vi "Settings Dialog.vi"(8 "error in (no error)":errorcluster, 11 "Settings in":T2={"Hardware Configuration"={"DAQmx Channel"="", "Max Input"=10.0, "Min Input"=-10.0, "Sample Rate"=1000.0, "DAQmx Task"=""}, "Logging Configuration"={"Log File Base Path"=path "", "TDMS File Reference"=refnum, "Samples to Save"=0, "Trigger - Time"=0, "Trigger - Threshold"=0.0, "Trigger - Channel"=0, "Enable Time Trigger"=FALSE, "Enable Threshold Trigger"=FALSE, "Always Log"=FALSE}, "MSpeed AO HW Config"={"MSpeed AO Channel"="", "Sample Rate(Hz)"=1000.0, "MSpeed AO Task"=""}, "Motor Config"={"VISA resource name"="", "Speed and Duration"=[{"Speed (%)"=10, "Duration (sec)"=120.0}, {"Speed (%)"=25, "Duration (sec)"=120.0}, {"Speed (%)"=50, "Duration (sec)"=120.0}]}, "2P Trigger Config"={"DO Line"="Dev1/port0/line0"}} {"Motor Config"."Speed and Duration"."Duration (sec)" min=0.0 max=100.0 step=0.1 format="%.1f"; "Motor Config"."Speed and Duration"."Speed (%)" min=0 max=100 step=1 format="%.1f"}) -> (0 "error out":errorcluster, 1 "Cancelled?":bool=TRUE, 2 "UI Refresh Needed?":bool, 3 "Settings out":T2={"Hardware Configuration"={"DAQmx Channel"="", "Max Input"=10.0, "Min Input"=-10.0, "Sample Rate"=1000.0, "DAQmx Task"=""}, "Logging Configuration"={"Log File Base Path"=path "C:/Users/jpassiak/Documents/LabVIEW Data/Logged Data.tdms", "TDMS File Reference"=refnum, "Samples to Save"=0, "Trigger - Time"=0, "Trigger - Threshold"=0.0, "Trigger - Channel"=0, "Enable Time Trigger"=FALSE, "Enable Threshold Trigger"=FALSE, "Always Log"=FALSE}, "MSpeed AO HW Config"={"MSpeed AO Channel"="", "Sample Rate(Hz)"=1000.0, "MSpeed AO Task"=""}, "Motor Config"={"VISA resource name"="", "Speed and Duration"=[{"Speed (%)"=10, "Duration (sec)"=120.0}, {"Speed (%)"=25, "Duration (sec)"=120.0}, {"Speed (%)"=50, "Duration (sec)"=120.0}]}, "2P Trigger Config"={"DO Line"="Dev1/port0/line0"}} {"Motor Config"."Speed and Duration"."Duration (sec)" min=0.0 max=100.0 step=0.1 format="%.1f"; "Motor Config"."Speed and Duration"."Speed (%)" min=0 max=100 step=1 format="%.1f"})   [LabVIEW 2016, in "Settings.lvlib"]
doc: "Dialog for selecting user specified settings."
uses:
  Settings.lvlib
  Settings.ctl
  Acquisition/Hardware Configuration.ctl
  Logging/Logging Configuration.ctl
  Motor Speed/MSpeed AO HW Config.ctl
  Motor Control/Motor Control Config.ctl
  Motor Control/Speed and Duration.ctl
  2P Trigger/2P Trigger Config.ctl
  <vilib>/Utility/xml.llb/Write to XML File(string).vi
  Acquisition/Acquisition.lvlib
  Logging/Logging.lvlib
  Motor Speed/Motor Speed AO.lvlib
  Motor Control/Motor Control.lvlib
  2P Trigger/2P Trigger.lvlib
panel:
  in  "Trigger Input DO Line":tag="Dev1/port0/line0"
  in  "VISA resource name":refnum<visa-resource-name>="COM3"
  in  "Speed and Duration":T1[](array[typedef])=[{"Speed (%)"=10, "Duration (sec)"=120.0}, {"Speed (%)"=25, "Duration (sec)"=120.0}, {"Speed (%)"=50, "Duration (sec)"=120.0}] {"Duration (sec)" min=0.0 max=100.0 step=0.1 format="%.1f"; "Speed (%)" min=0 max=100 step=1 format="%.1f"}
  in  "MSpeed Sample Rate":dbl=1000.0
  in  "MSpeed AO Channel":tag="Dev2/ao0"
  in  "Log when triggered":bool
  in  "Trigger Channel":u32
  in  "Samples to Log":u32=500 min=1
  in  "Trigger Threshold (V)":dbl=2.0
  in  "Trigger Time (min)":u32=1
  in  "Enable Threshold Trigger (V):":bool
  in  "Enable Time Trigger (min):":bool
  in  "Always Log":bool=TRUE
  in  "Sample Rate":dbl=1000.0
  in  "Minimum Input":dbl=-10.0
  in  "Maximum Input":dbl=10.0
  in  "DAQmx Channel":tag="Dev1/ai0"
  in  "Log File Path":path
  in  "Cancel Button":bool
  in  "OK Button":bool
  # "Acquisition"
  # "Motor"
  # "Non visible portion of dialog (needed for connector pane)."
  # "Speed (%)"
  # "Duration (sec)"
  # "Trigger"
  # "Speed monitor"
  # "2P trigger"
  # "Logging"
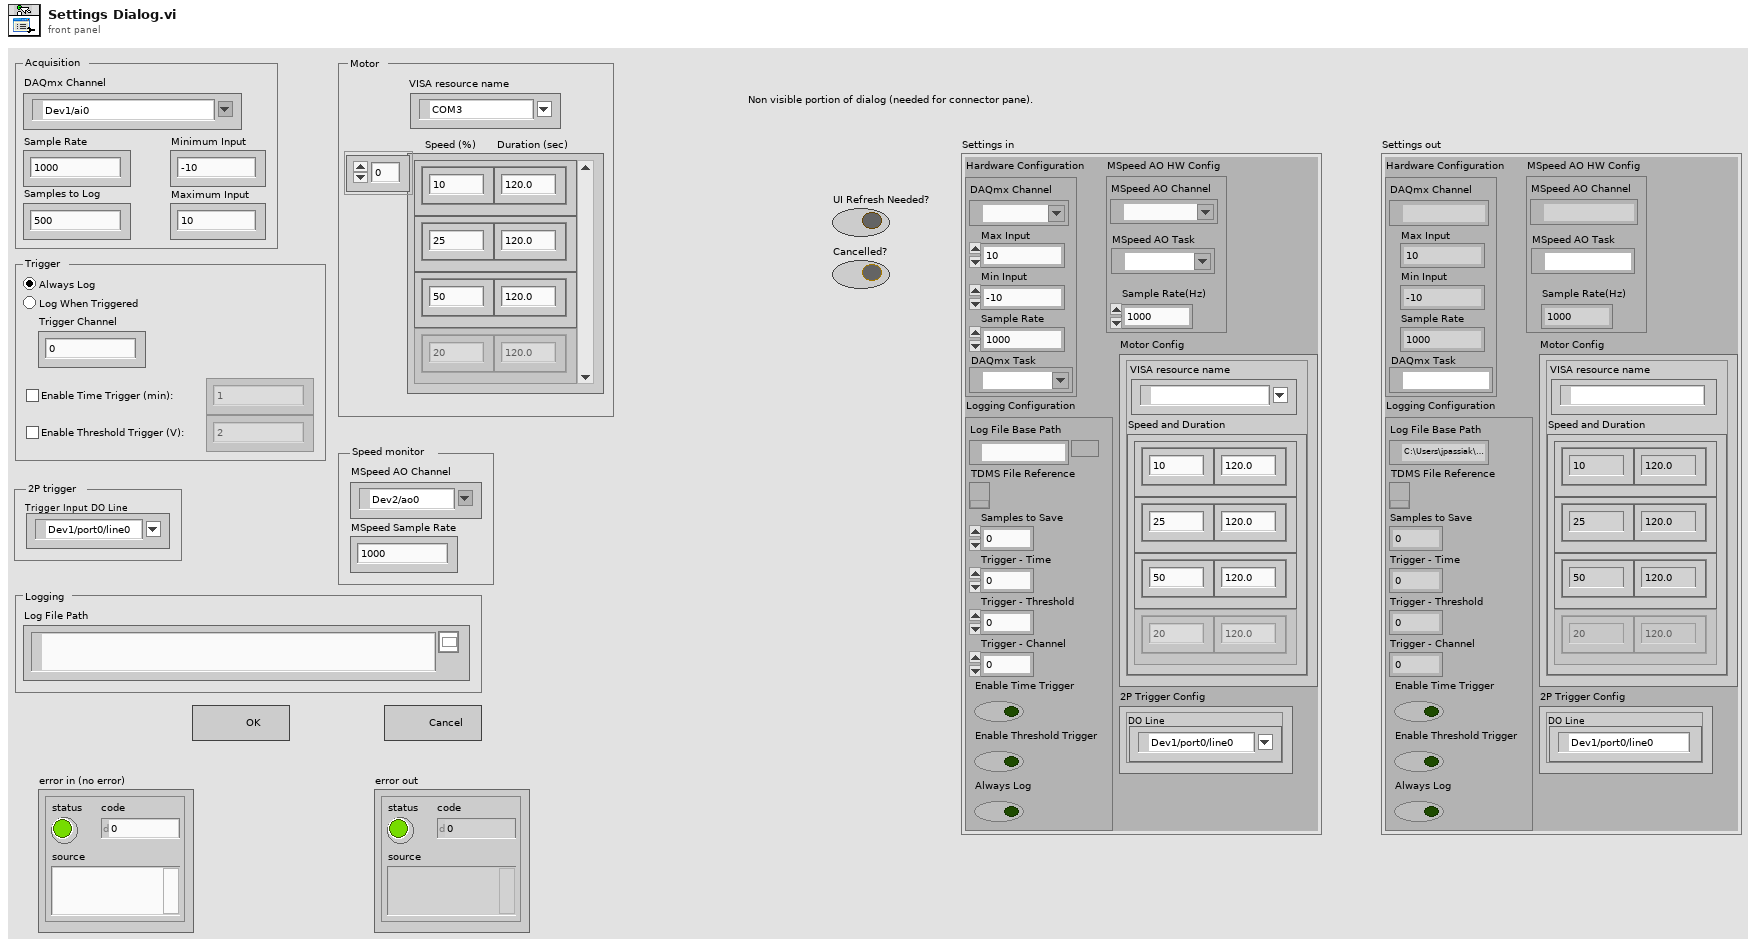
[diagram p1: front panel]
types:
  T1 = typedef "Motor Control.lvlib/Speed and Duration.ctl" = cluster{"Speed (%)":i32, "Duration (sec)":dbl}
  T2 = typedef "Settings.lvlib/Settings.ctl" = cluster{"Hardware Configuration":T3, "Logging Configuration":T4, "MSpeed AO HW Config":T5, "Motor Config":T6, "2P Trigger Config":T7}
  T3 = typedef "Acquisition.lvlib/Hardware Configuration.ctl" = cluster{"DAQmx Channel":tag, "Max Input":dbl, "Min Input":dbl, "Sample Rate":dbl, "DAQmx Task":refnum<k21>}
  T4 = typedef "Logging.lvlib/Logging Configuration.ctl" = cluster{"Log File Base Path":path, "TDMS File Reference":refnum<k34>, "Samples to Save":u32, "Trigger - Time":u32, "Trigger - Threshold":dbl, "Trigger - Channel":u32, "Enable Time Trigger":bool, "Enable Threshold Trigger":bool, "Always Log":bool}
  T5 = typedef "Motor Speed AO.lvlib/MSpeed AO HW Config.ctl" = cluster{"MSpeed AO Channel":tag, "Sample Rate(Hz)":dbl, "MSpeed AO Task":refnum<k21>}
  T6 = typedef "Motor Control.lvlib/Motor Control Config.ctl" = cluster{"VISA resource name":refnum<visa-resource-name>, "Speed and Duration":T1[]}
  T7 = typedef "2P Trigger.lvlib/2P Trigger Config.ctl" = cluster{"DO Line":tag}
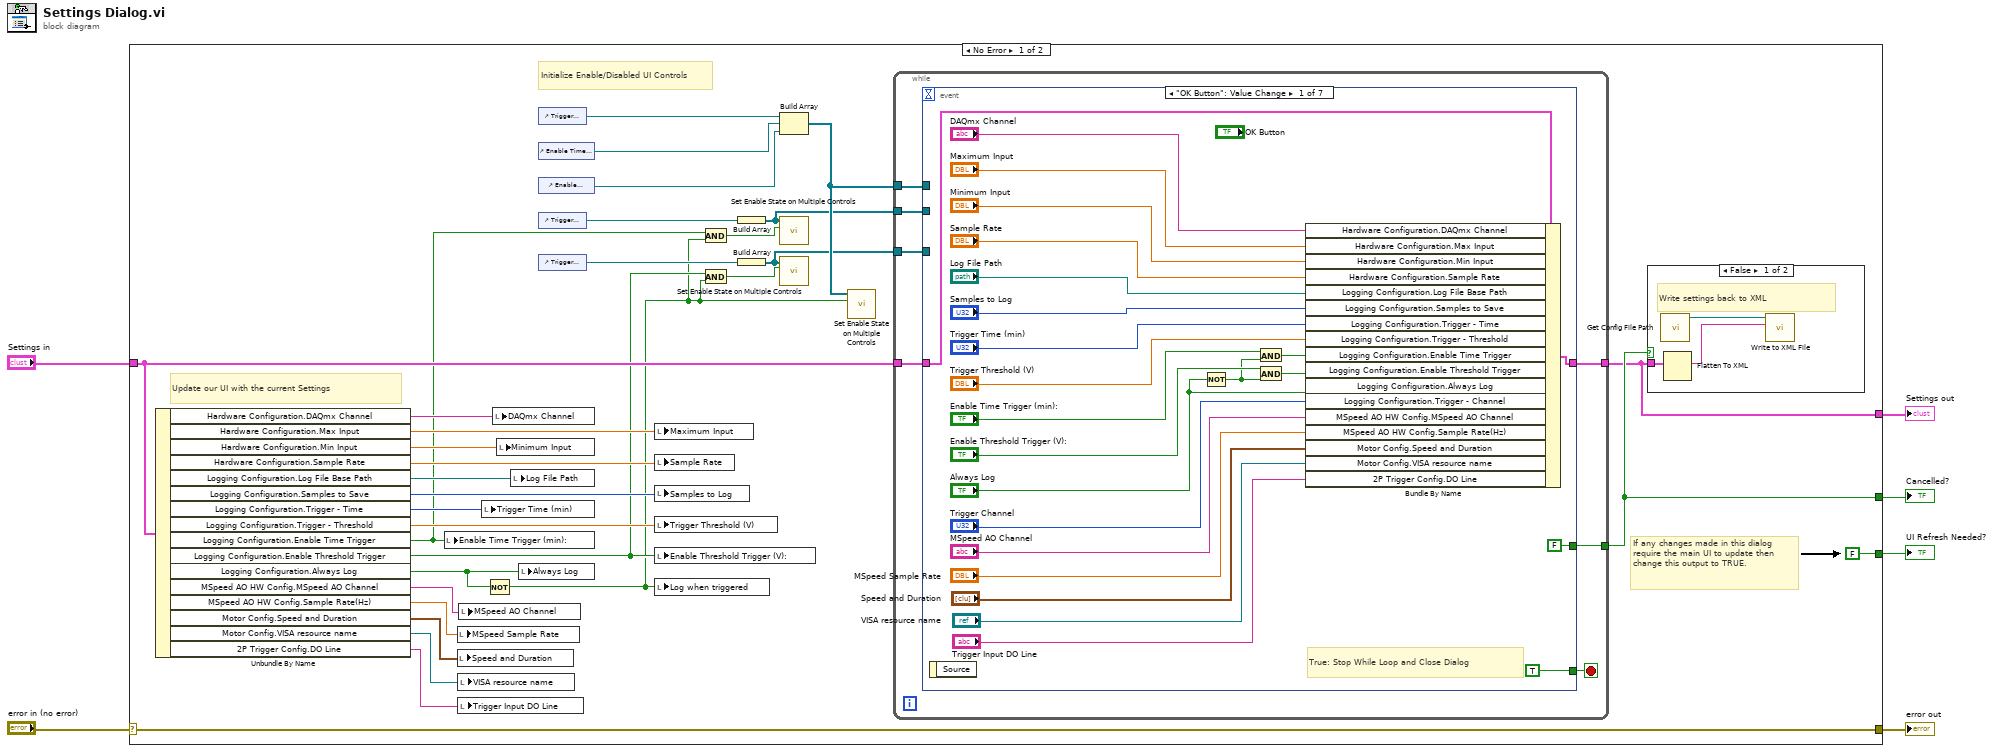
[diagram p0: block diagram]
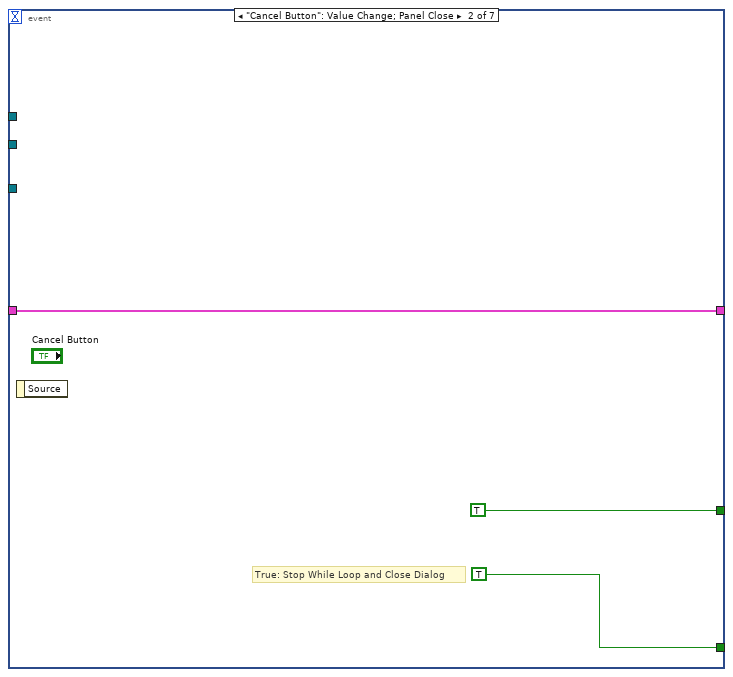
[diagram p2: hidden frame]
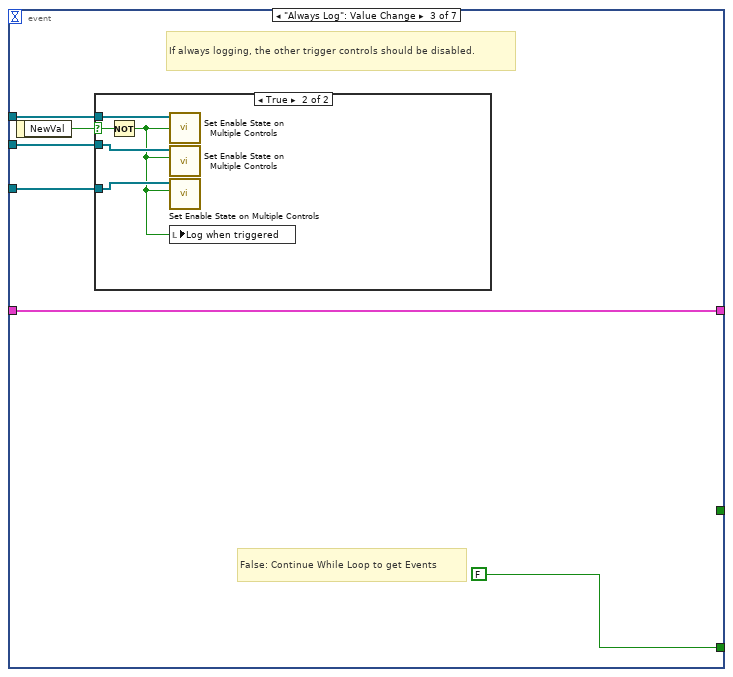
[diagram p3: hidden frame]
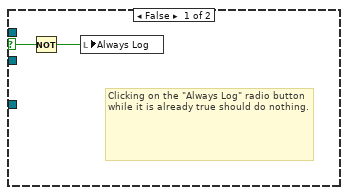
[diagram p4: hidden frame]
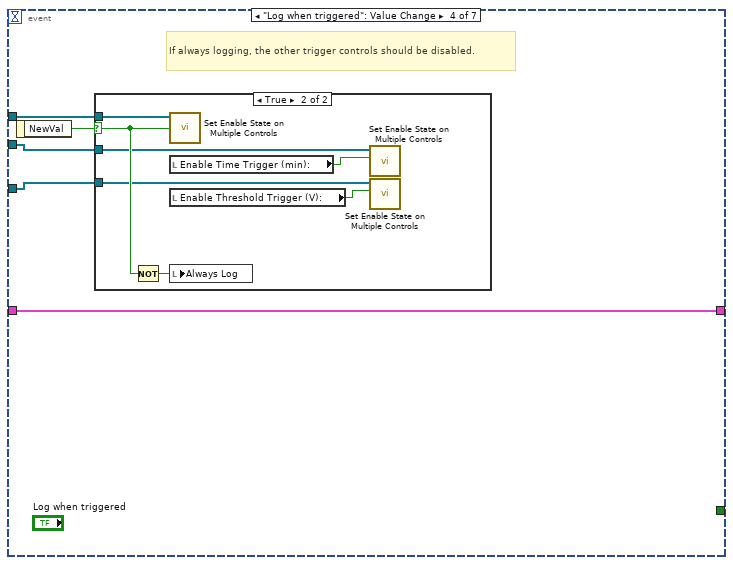
[diagram p5: hidden frame]
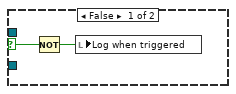
[diagram p6: hidden frame]
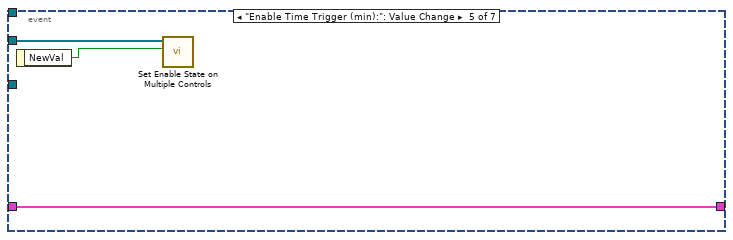
[diagram p7: hidden frame]
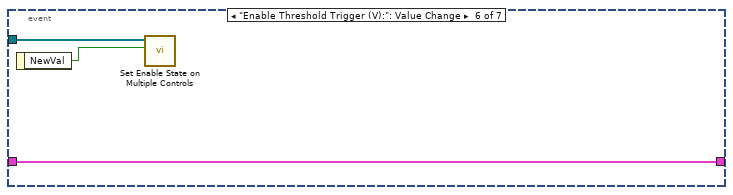
[diagram p8: hidden frame]
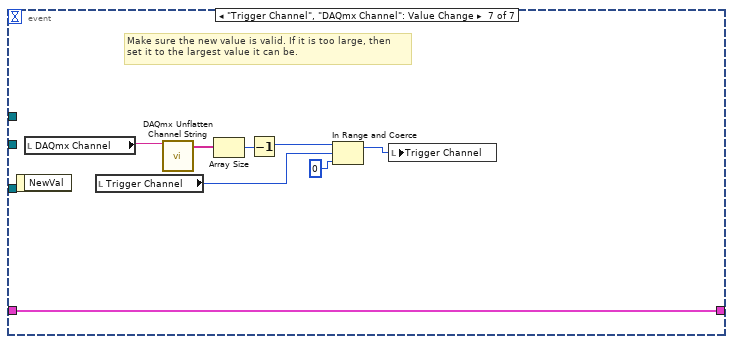
[diagram p9: hidden frame]
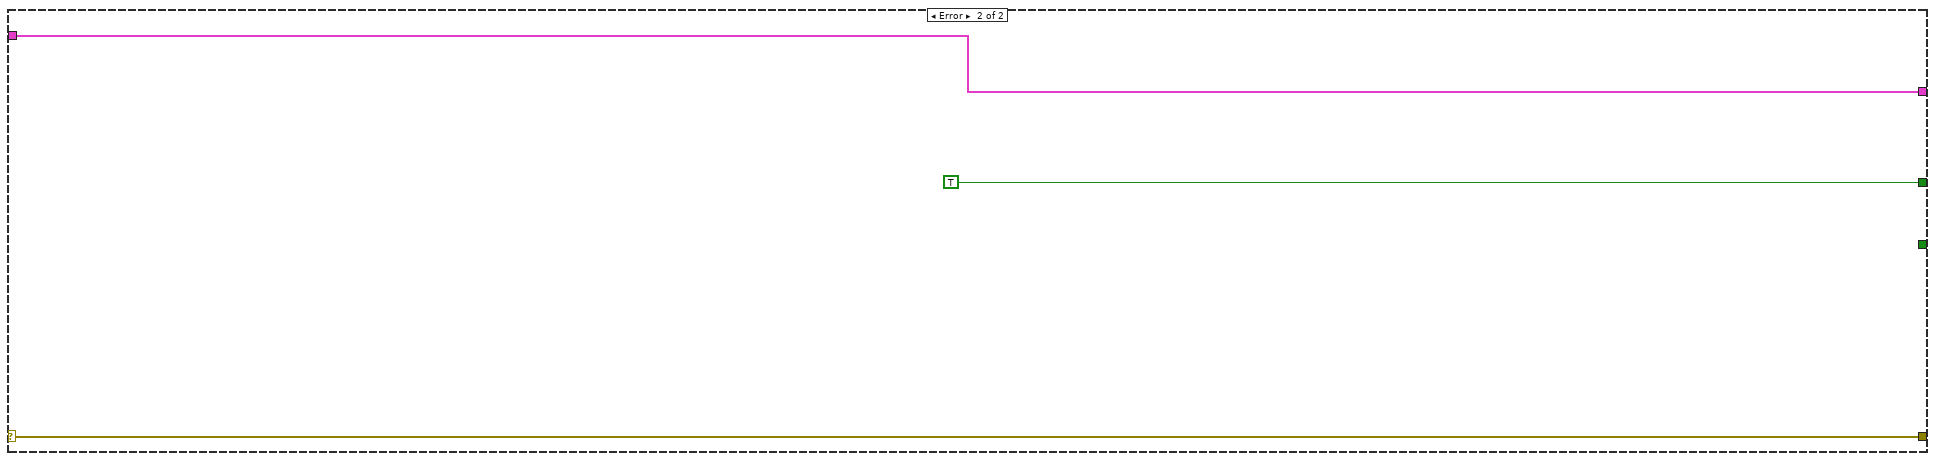
[diagram p11: hidden frame]
diagram:
  n1 = case shown="No Error" "error in (no error)" {
    selector: "error in (no error)" -> [w38 w119]
    tunnel: [w38 w119] -> w6
    tunnel: "Settings in" -> [w24 w118]
    tunnel: [w35 w118] -> w4
    tunnel: [FALSE ("UI Refresh Needed?") _] -> w3
    tunnel: [w36 TRUE ("UI Refresh Needed?")] -> w2
    frame No Error {
      # "Update our UI with the current Settings"
      # "Initialize Enable/Disabled UI Controls"
      # "If any changes made in this dialog require the main UI to update then change this output to TRUE."
      n2 = Unbundle By Name(w24) -> ("Hardware Configuration.DAQmx Channel"=w31:tag, "Hardware Configuration.Max Input"=w32:dbl, "Hardware Configuration.Min Input"=w33:dbl, "Hardware Configuration.Sample Rate"=w34:dbl, "Logging Configuration.Log File Base Path"=w30:path, "Logging Configuration.Samples to Save"=w29:u32, "Logging Configuration.Trigger - Time"=w28:u32, "Logging Configuration.Trigger - Threshold"=w27:dbl, "Logging Configuration.Enable Time Trigger"=w16:bool, "Logging Configuration.Enable Threshold Trigger"=w15:bool, "Logging Configuration.Always Log"=w26:bool, "MSpeed AO HW Config.MSpeed AO Channel"=w11:tag, "MSpeed AO HW Config.Sample Rate(Hz)"=w10:dbl, "Motor Config.Speed and Duration"=w9:T1[], "Motor Config.VISA resource name"=w8:refnum<visa-resource-name>, "2P Trigger Config.DO Line"=w7:tag)
      n3 = local write "Enable Time Trigger (min):"(w16) -> ()
      n4 = local write "MSpeed Sample Rate"(w10) -> ()
      n5 = local write "Speed and Duration"(w9) -> ()
      n6 = local write "VISA resource name"(w8) -> ()
      n7 = local write "Trigger Input DO Line"(w7) -> ()
      n8 = local write "MSpeed AO Channel"(w11) -> ()
      n9 = local write "Trigger Time (min)"(w28) -> ()
      n10 = Not(x=w26) -> (.not. x?=w12:bool)
      n11 = local write "DAQmx Channel"(w31) -> ()
      n12 = local write "Minimum Input"(w33) -> ()
      n13 = local write "Log File Path"(w30) -> ()
      n14 = local write "Always Log"(w26) -> ()
      n15 = control-ref of="Trigger Channel"() -> (w23:refnum<vi>)
      n16 = control-ref of="Enable Time Trigger (min):"() -> (w22:refnum<vi>)
      n17 = control-ref of="Enable Threshold Trigger (V):"() -> (w21:refnum<vi>)
      n18 = control-ref of="Trigger Time (min)"() -> (w20:refnum<vi>)
      n19 = control-ref of="Trigger Threshold (V)"() -> (w19:refnum<vi>)
      n20 = local write "Maximum Input"(w32) -> ()
      n21 = local write "Sample Rate"(w34) -> ()
      n22 = local write "Samples to Log"(w29) -> ()
      n23 = local write "Trigger Threshold (V)"(w27) -> ()
      n24 = local write "Enable Threshold Trigger (V):"(w15) -> ()
      n25 = local write "Log when triggered"(w12) -> ()
      n26 = And(x=w16, y=w12) -> (x .and. y?=w18:bool)
      n27 = And(x=w15, y=w12) -> (x .and. y?=w17:bool)
      n28 = Build Array(w20) -> (w14:refnum<vi>[])
      n29 = Build Array(w19) -> (w13:refnum<vi>[])
      n30 = Build Array(w23, w22, w21) -> (w25:refnum<vi>[])
      n31 = call "Set Enable State on Multiple Controls.vi"("Enable?"=w18, "Controls"=w14) -> ()  [unwired: 10 in]
      n32 = call "Set Enable State on Multiple Controls.vi"("Enable?"=w17, "Controls"=w13) -> ()  [unwired: 10 in]
      n33 = call "Set Enable State on Multiple Controls.vi"("Enable?"=w12, "Controls"=w25) -> ()  [unwired: 10 in]
      n34 = while {
        tunnel: [w45] -> w36
        tunnel: [w44] -> w35
        tunnel: w24 -> [w43]
        tunnel: w25 -> [w41]
        tunnel: w14 -> [w40]
        tunnel: w13 -> [w39]
        stop <- w42 stop-if-true
        n35 = event shown="[0] \"OK Button\": Value Change" {
          selector: _ -> [_ _ _ _ _ _ _]
          dyn-events: _ -> [_ _ _ _ _ _ _]
          timeout: _ -> [_ _ _ _ _ _ _]
          tunnel: [w67 w72 w78 w90 w102 w105 w113] -> w44
          tunnel: w43 -> [w66 w72 w78 w90 w102 w105 w113]
          tunnel: [FALSE ("UI Refresh Needed?") TRUE ("UI Refresh Needed?") _ _ _ _ _] -> w45
          tunnel: [TRUE TRUE FALSE _ _ _ _] -> w42
          tunnel: w41 -> [_ _ w76 w89 _ _ _]
          tunnel: w40 -> [_ _ w74 w87 w101 _ _]
          tunnel: w39 -> [_ _ w73 w86 _ w104 _]
          event "OK Button": Value Change {
            # "True: Stop While Loop and Close Dialog"
            n36 = event-data() -> ()  [unwired: 1 in, 1 out]
            n37 = Not(x="Always Log") -> (.not. x?=w51:bool)
            n38 = And(x="Enable Time Trigger (min):", y=w51) -> (x .and. y?=w52:bool)
            n39 = And(x="Enable Threshold Trigger (V):", y=w51) -> (x .and. y?=w54:bool)
            n40 = Bundle By Name(cluster=w66, "Hardware Configuration.DAQmx Channel"="DAQmx Channel", "Hardware Configuration.Max Input"="Maximum Input", "Hardware Configuration.Min Input"="Minimum Input", "Hardware Configuration.Sample Rate"="Sample Rate", "Logging Configuration.Log File Base Path"="Log File Path", "Logging Configuration.Samples to Save"="Samples to Log", "Logging Configuration.Trigger - Time"="Trigger Time (min)", "Logging Configuration.Trigger - Threshold"="Trigger Threshold (V)", "Logging Configuration.Enable Time Trigger"=w52, "Logging Configuration.Enable Threshold Trigger"=w54, "Logging Configuration.Always Log"="Always Log", "Logging Configuration.Trigger - Channel"="Trigger Channel", "MSpeed AO HW Config.MSpeed AO Channel"="MSpeed AO Channel", "MSpeed AO HW Config.Sample Rate(Hz)"="MSpeed Sample Rate", "Motor Config.Speed and Duration"="Speed and Duration", "Motor Config.VISA resource name"="VISA resource name", "2P Trigger Config.DO Line"="Trigger Input DO Line") -> (w67:T2)
          }
          event "Cancel Button": Value Change; Panel Close {
            # "True: Stop While Loop and Close Dialog"
            n41 = event-data() -> ()  [unwired: 1 in, 1 out]
          }
          event "Always Log": Value Change {
            # "False: Continue While Loop to get Events"
            # "If always logging, the other trigger controls should be disabled."
            n42 = event-data() -> ("NewVal"=w75:bool)  [unwired: 1 in]
            n43 = case shown="True" w75 {
              selector: w75 -> [w80 w85]
              tunnel: w76 -> [_ w84]
              tunnel: w74 -> [_ w83]
              tunnel: w73 -> [_ w82]
              frame False {
                # "Clicking on the \"Always Log\" radio button while it is already true should do nothing."
                n44 = Not(x=w80) -> (.not. x?=w79:bool)
                n45 = local write "Always Log"(w79) -> ()
              }
              frame True {
                n46 = Not(x=w85) -> (.not. x?=w81:bool)
                n47 = call "Set Enable State on Multiple Controls.vi"("Enable?"=w81, "Controls"=w84) -> ()  [unwired: 10 in]
                n48 = call "Set Enable State on Multiple Controls.vi"("Enable?"=w81, "Controls"=w83) -> ()  [unwired: 10 in]
                n49 = call "Set Enable State on Multiple Controls.vi"("Enable?"=w81, "Controls"=w82) -> ()  [unwired: 10 in]
                n50 = local write "Log when triggered"(w81) -> ()
              }
            }
          }
          event "Log when triggered": Value Change {
            # "If always logging, the other trigger controls should be disabled."
            n51 = event-data() -> ("NewVal"=w88:bool)  [unwired: 1 in]
            n52 = case shown="True" w88 {
              selector: w88 -> [w92 w98]
              tunnel: w89 -> [_ w99]
              tunnel: w87 -> [_ w96]
              tunnel: w86 -> [_ w95]
              frame False {
                n53 = Not(x=w92) -> (.not. x?=w91:bool)
                n54 = local write "Log when triggered"(w91) -> ()
              }
              frame True {
                n55 = Not(x=w98) -> (.not. x?=w97:bool)
                n56 = call "Set Enable State on Multiple Controls.vi"("Enable?"=w98, "Controls"=w99) -> ()  [unwired: 10 in]
                n57 = local read "Enable Time Trigger (min):"() -> (w93:bool)
                n58 = local read "Enable Threshold Trigger (V):"() -> (w94:bool)
                n59 = local write "Always Log"(w97) -> ()
                n60 = call "Set Enable State on Multiple Controls.vi"("Enable?"=w93, "Controls"=w96) -> ()  [unwired: 10 in]
                n61 = call "Set Enable State on Multiple Controls.vi"("Enable?"=w94, "Controls"=w95) -> ()  [unwired: 10 in]
              }
            }
          }
          event "Enable Time Trigger (min):": Value Change {
            n62 = event-data() -> ("NewVal"=w100:bool)  [unwired: 1 in]
            n63 = call "Set Enable State on Multiple Controls.vi"("Enable?"=w100, "Controls"=w101) -> ()  [unwired: 10 in]
          }
          event "Enable Threshold Trigger (V):": Value Change {
            n64 = event-data() -> ("NewVal"=w103:bool)  [unwired: 1 in]
            n65 = call "Set Enable State on Multiple Controls.vi"("Enable?"=w103, "Controls"=w104) -> ()  [unwired: 10 in]
          }
          event "Trigger Channel", "DAQmx Channel": Value Change {
            # "Make sure the new value is valid. If it is too large, then\nset it to the largest value it can be."
            n66 = event-data() -> ()  [unwired: 1 in, 1 out]
            n67 = local read "DAQmx Channel"() -> (w112:tag)
            n68 = local read "Trigger Channel"() -> (w106:u32)
            n69 = call <vilib>:"DAQmx Unflatten Channel String.vi"("names in"=w112) -> ("names out"=w111:string[])  [unwired: 13 in, 1 out]
            n70 = Array Size(array=w111) -> (size(s)=w110:i32)
            n71 = Decrement(x=w110) -> (x-1=w109:i32)
            n72 = In Range and Coerce(upper limit=w109, x=w106, lower limit=u32 0) -> (coerced(x)=w107:u32)  [unwired: 1 out]
            n73 = local write "Trigger Channel"(w107) -> ()
          }
        }
      }
      n74 = case shown="False" w36 {
        tunnel: w35 -> [w115 _]
        frame False {
          # "Write settings back to XML"
          n75 = call "Get Config File Path.vi"() -> ("XML File Path"=w116:path)  [unwired: 10 in, 1 out]
          n76 = Flatten To XML(anything=w115) -> (xml string=w114:string)
          n77 = call-poly <vilib>:"Write to XML File.vi"("XML Input"=w114, "XML File Path"=w116) -> ()  [unwired: 7 in, 3 out]
        }
        frame True {
        }
      }
    }
    frame Error {
    }
  }
  "UI Refresh Needed?" <- w3
  "error out" <- w6
  "Settings out" <- w4
  "Cancelled?" <- w2
